vi "函数类型1测试.vi"() -> ()   [LabVIEW 2010]
uses:
  全局量/试验配置信息.vi
panel:
  out "D_IN_1":string[][](table) caption="表格"
  in  "加载文件名称":string
  out "配置文件路径":path
  out "配置文件目录":path
  in  "加载配置文件列表":u16(ring)
  in  "同步_1":i32
  in  "数组_反馈值":dbl[][](array[numeric])
  in  "第几个数据":i32
  in  "第几组数据":i32
  in  "数组_设定值":dbl[][](array[numeric])
  in  "数组_选择":bool[](array[boolean])
  out "light_32":bool
  out "light_31":bool
  out "light_30":bool
  out "light_29":bool
  out "light_28":bool
  out "light_27":bool
  out "light_26":bool
  out "light_25":bool
  out "light_24":bool
  out "light_23":bool
  out "light_22":bool
  out "light_21":bool
  out "light_20":bool
  out "light_19":bool
  out "light_18":bool
  out "light_17":bool
  out "Analog_back":string[][](table) caption="表格"
  in  "A_32":bool
  in  "A_31":bool
  in  "A_30":bool
  in  "A_29":bool
  in  "A_28":bool
  in  "A_27":bool
  in  "A_26":bool
  in  "A_25":bool
  in  "A_24":bool
  in  "A_23":bool
  in  "A_22":bool
  in  "A_21":bool
  in  "A_20":bool
  in  "A_19":bool
  in  "A_18":bool
  in  "A_17":bool
  out "合格？":bool[][](array[boolean])
  out "测试结论":string
  out "light_16":bool
  out "light_15":bool
  out "light_14":bool
  out "light_13":bool
  out "light_12":bool
  out "light_11":bool
  out "light_10":bool
  out "light_9":bool
  out "light_8":bool
  out "light_7":bool
  out "light_6":bool
  out "light_5":bool
  out "light_4":bool
  out "light_3":bool
  out "light_2":bool
  out "light_1":bool
  out "退出？":bool
  in  "btn_反选":bool
  in  "btn_全选":bool
  in  "A_16":bool
  in  "A_15":bool
  in  "A_14":bool
  in  "A_13":bool
  in  "A_12":bool
  in  "A_11":bool
  in  "A_10":bool
  in  "A_9":bool
  in  "A_8":bool
  in  "A_7":bool
  in  "A_6":bool
  in  "A_5":bool
  in  "A_4":bool
  in  "A_3":bool
  in  "A_2":bool
  in  "A_1":bool
  in  "btn_取消":bool
  in  "btn_开始测试":bool
  in  "Analog_IN":string[][](table) caption="表格"
  out "Analog_WC":string[][](table) caption="表格"
  # "模拟量选择及输入值（V）"
  # "模拟量反馈值（V）"
  # "模拟量误差值（%）"
  # "加载配置文件："
  # "测试结论："
  # "从0开始"
  # "从1开始,第0列没有使用"
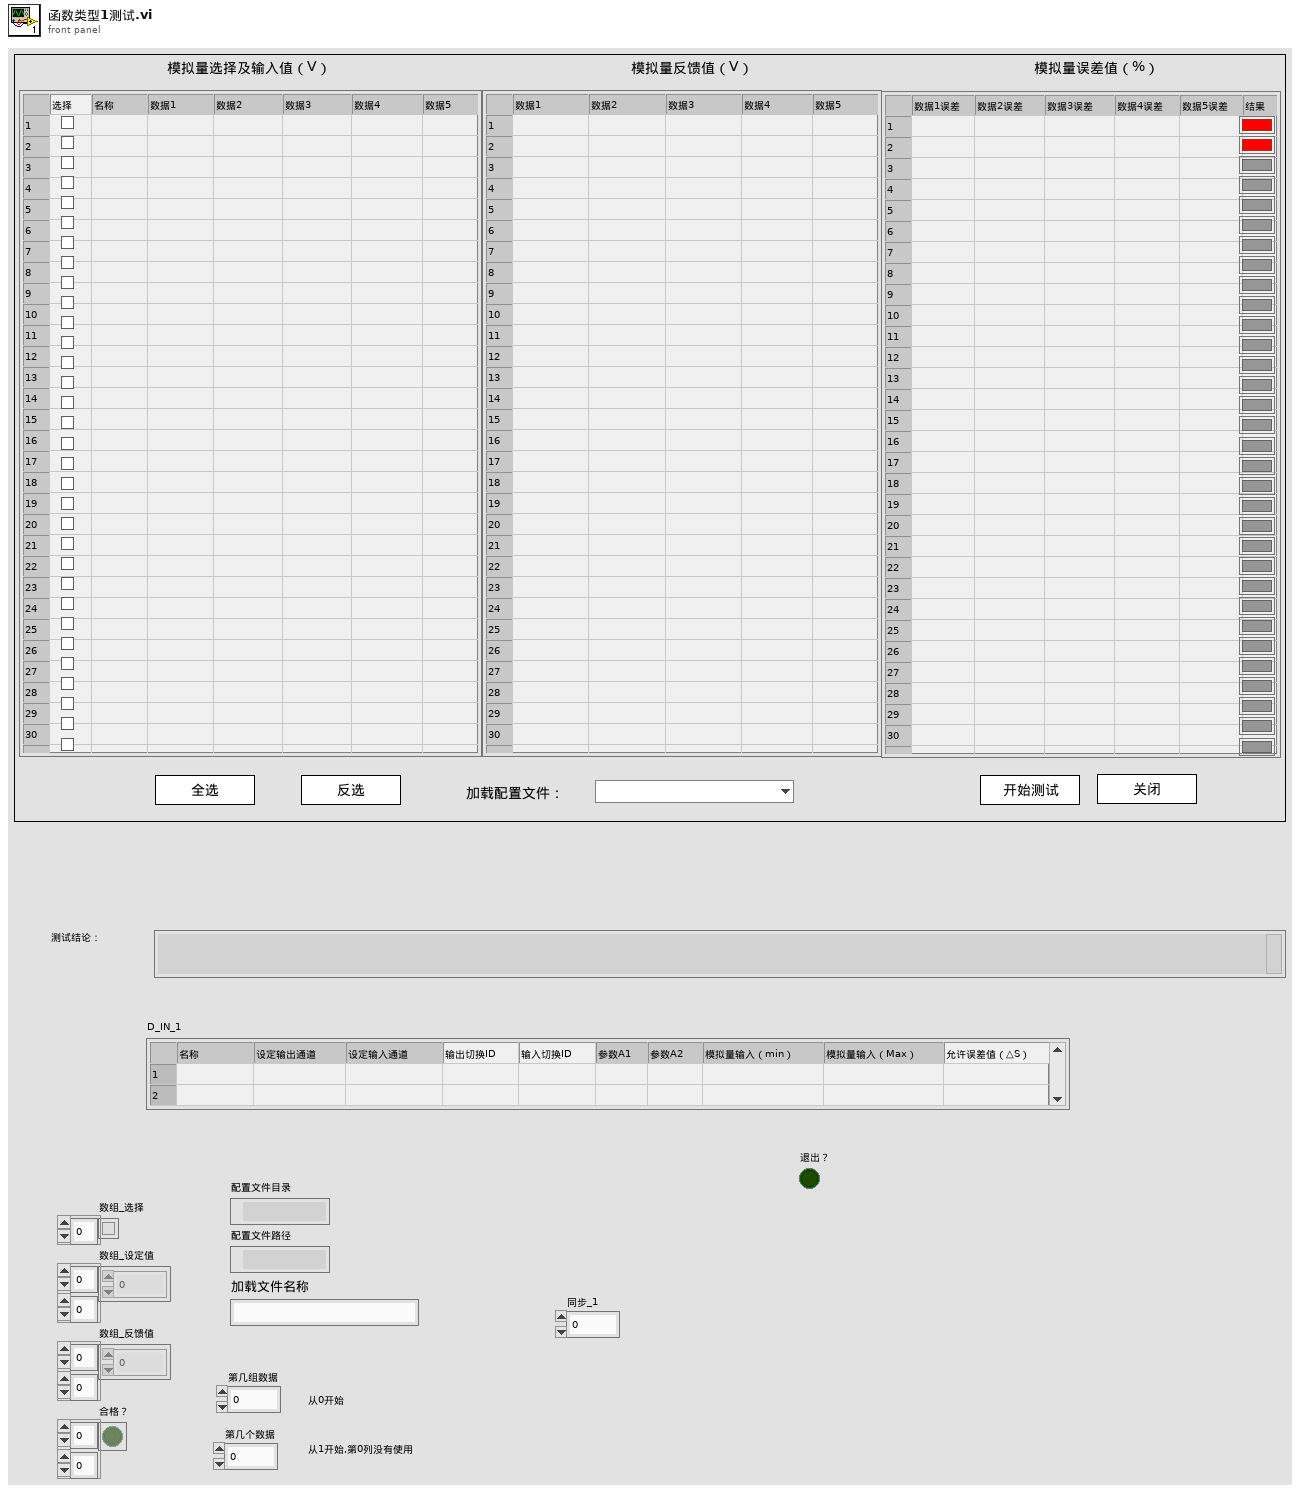
[diagram p1: front panel]
types:
  T1 = enum8{"Enabled", "Disabled", "Disabled and Grayed Out"}
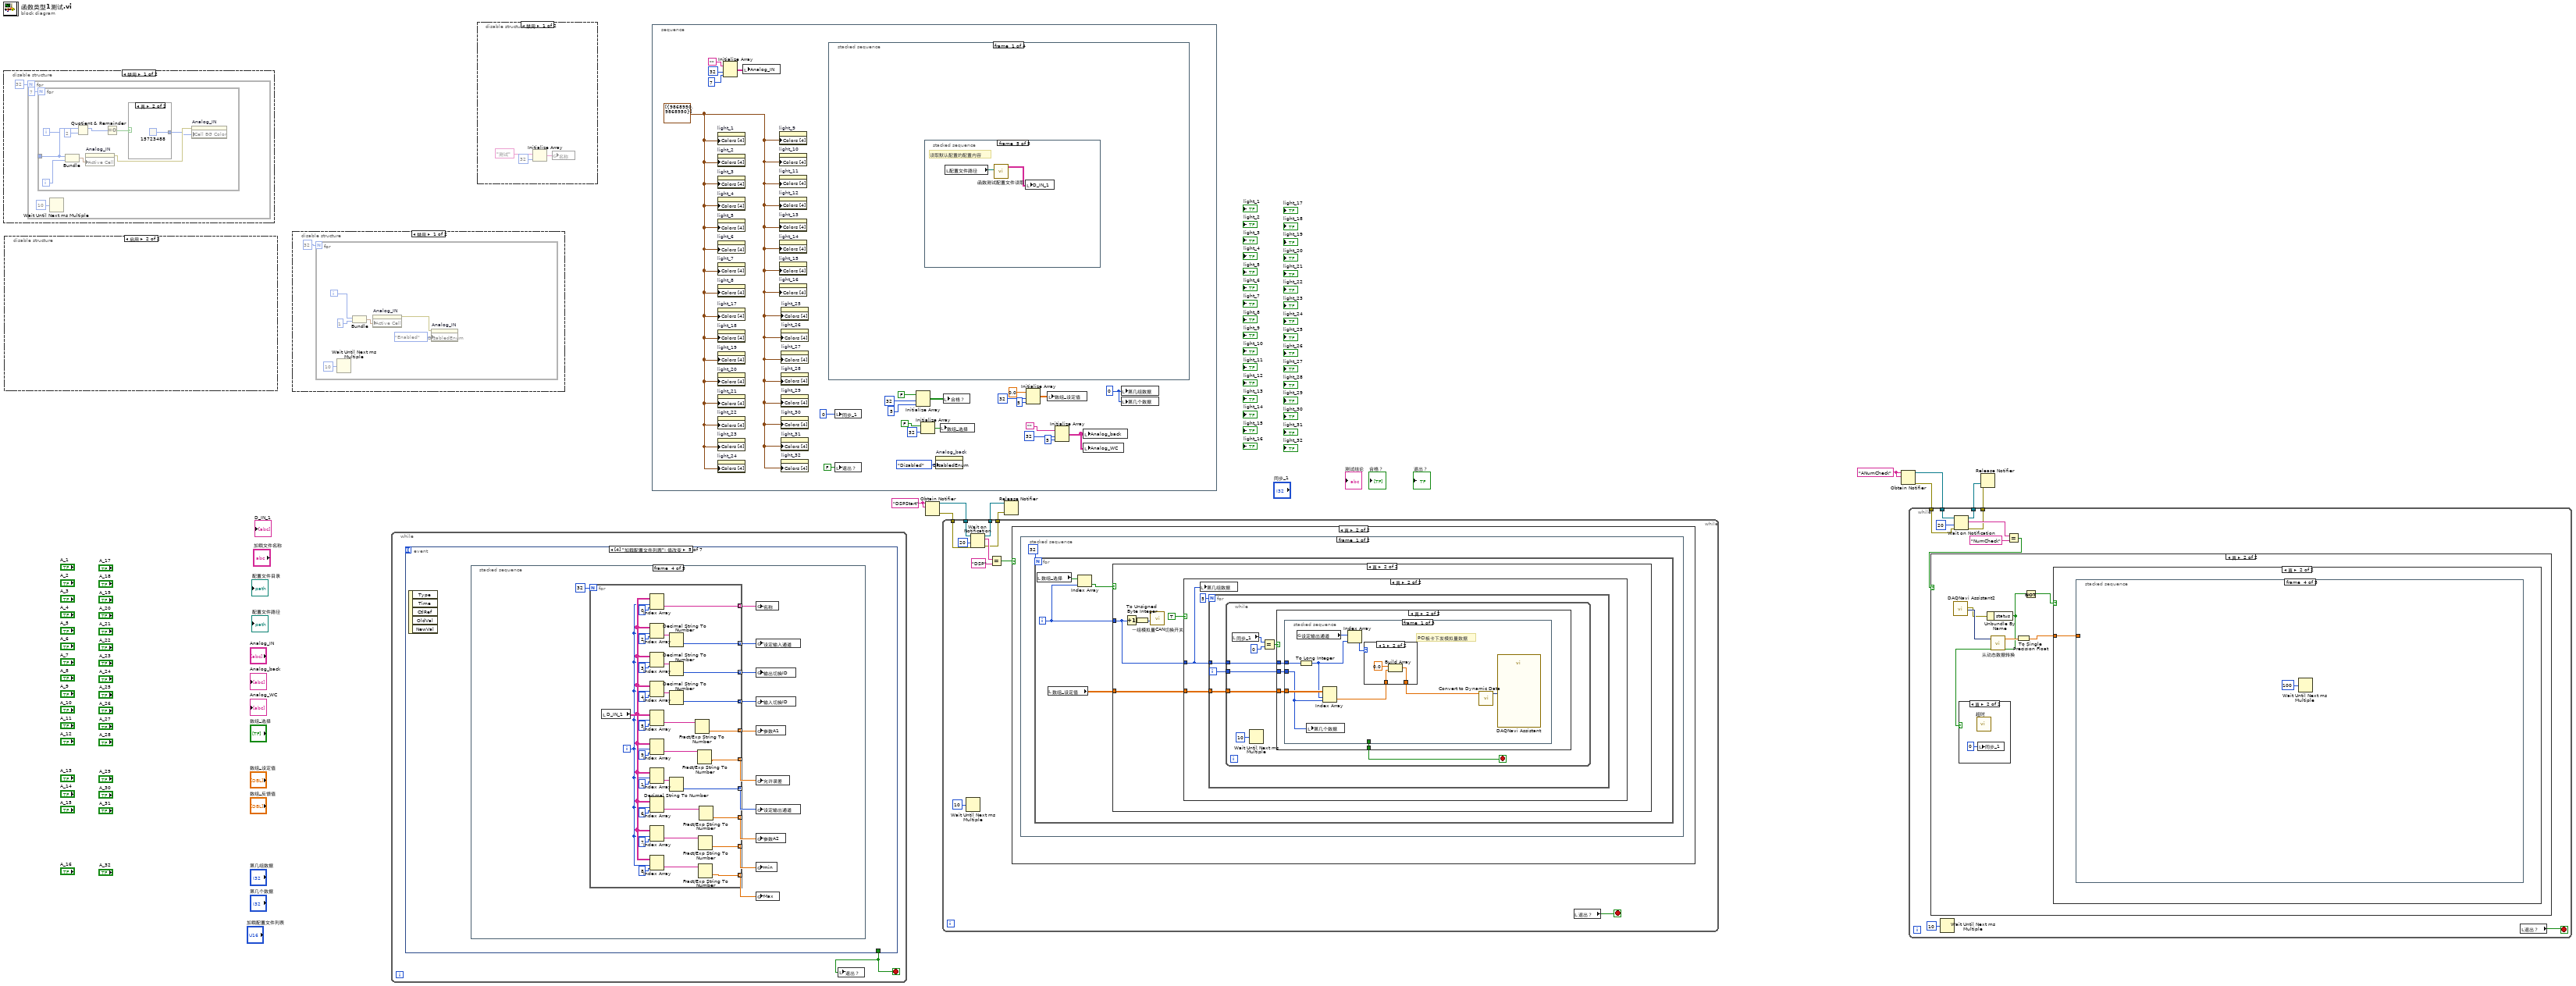
[diagram p0: block diagram]
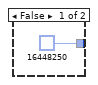
[diagram p3: hidden frame]
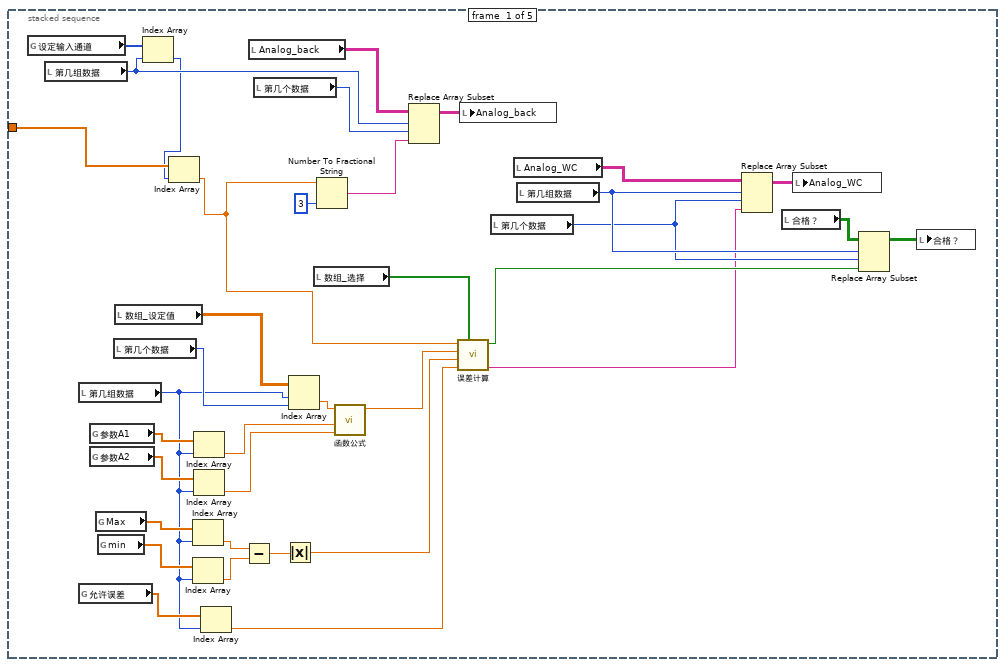
[diagram p8: hidden frame]
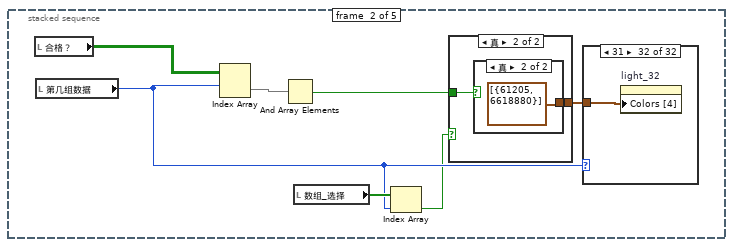
[diagram p9: hidden frame]
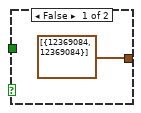
[diagram p10: hidden frame]
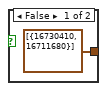
[diagram p11: hidden frame]
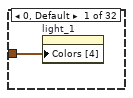
[diagram p12: hidden frame]
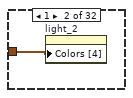
[diagram p13: hidden frame]
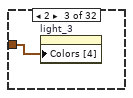
[diagram p14: hidden frame]
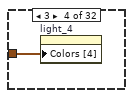
[diagram p15: hidden frame]
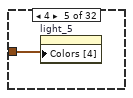
[diagram p16: hidden frame]
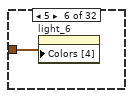
[diagram p17: hidden frame]
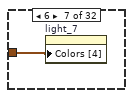
[diagram p18: hidden frame]
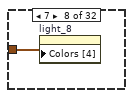
[diagram p19: hidden frame]
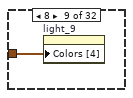
[diagram p20: hidden frame]
diagram:
  w5 = "ANumCheck" ("名称（未命名）")
  w8 = "DSPStart" ("名称（未命名）")
  n1 = disable-structure shown="禁用" {
    frame Disabled {
      n2 = for {
        N: 32 -> [_]
        i -> [w13]
        n3 = for {
          N: 7 -> [_]
          tunnel: w13 -> [w21]
          i -> [w15]
          n4 = Bundle(w21, w15) -> (w18:cluster{i32, i32})  [unwired: 1 in]
          n5 = Quotient & Remainder(x=w21, y=2) -> (x-y*floor(x/y)=w19:i32)  [unwired: 1 out]
          n6 = property on="Analog_IN" class="Tbl (严格)"("Active Cell"=w18) -> (error out=w17:errorcluster)  [unwired: 2 in, 1 out]
          n7 = Equal To 0?(x=w19) -> (x = 0?=w22:bool)
          n8 = case shown="真" w22 {
            tunnel: [u32 16448250 u32 15723488] -> w16
            frame False {
            }
            frame True {
            }
          }
          n9 = property on="Analog_IN" class="Tbl (严格)"(error in=w17, "Cell BG Color"=w16) -> ()  [unwired: 1 in, 2 out]
        }
        n10 = Wait Until Next ms Multiple(millisecond multiple=u32 10 ("毫秒倍数")) -> ()  [unwired: 1 out]
      }
    }
    frame Enabled {
    }
  }
  n11 = disable-structure shown="启用" {
    frame Disabled {
      n12 = for {
        N: 32 -> [_]
        i -> [w26]
        n13 = for {
          N: 7 -> [_]
          tunnel: w26 -> [w29]
          i -> [w30]
          n14 = Bundle(w29, w30) -> (w33:cluster{i32, i32})  [unwired: 1 in]
          n15 = property on="Analog_IN" class="Tbl (严格)"("Active Cell"=w33) -> (error out=w31:errorcluster)  [unwired: 2 in, 1 out]
          n16 = property on="Analog_IN" class="Tbl (严格)"(error in=w31, "Justify"=enum16{"Left", "Center", "Right"}."Left" ("活动单元格:单元格对齐")) -> ()  [unwired: 1 in, 2 out]
        }
        n17 = Wait Until Next ms Multiple(millisecond multiple=u32 10 ("毫秒倍数")) -> ()  [unwired: 1 out]
      }
    }
    frame Enabled {
    }
  }
  n18 = disable-structure shown="禁用" {
    frame Disabled {
      n19 = for {
        N: 32 -> [_]
        i -> [w39]
        n20 = Wait Until Next ms Multiple(millisecond multiple=u32 10 ("毫秒倍数")) -> ()  [unwired: 1 out]
        n21 = Bundle(w39, 1) -> (w38:cluster{i32, i32})  [unwired: 1 in]
        n22 = property on="Analog_IN" class="Tbl (严格)"("Active Cell"=w38) -> (error out=w35:errorcluster)  [unwired: 2 in, 1 out]
        n23 = property on="Analog_IN" class="Tbl (严格)"(error in=w35, "DisabledEnum"=T1."Enabled" ("禁用")) -> ()  [unwired: 1 in, 2 out]
      }
    }
    frame Enabled {
    }
  }
  n24 = while {
    stop <- w41 stop-if-true
    n25 = event shown="[4] \"加载配置文件列表\": 值改变" {
      selector: _ -> [_ _ _ _ _ _ _]
      dyn-events: _ -> [_ _ _ _ _ _ _]
      timeout: _ -> [_ _ _ _ _ _ _]
      tunnel: [_ TRUE TRUE _ _ _ _] -> w41
      event Timeout {
        n26 = event-data() -> ()  [unwired: 1 in, 2 out]
      }
      event Panel Close {
        n27 = event-data() -> ()  [unwired: 1 in, 3 out]
      }
      event "btn_取消": Value Change {
        n28 = event-data() -> ()  [unwired: 1 in, 5 out]
      }
      event "btn_开始测试": Value Change {
        n29 = event-data() -> ()  [unwired: 1 in, 5 out]
        n30 = stacked-sequence {
          frame #0 {
            w49 = 0 ("第几组数据")
            # "测试期间不准退出防止程序卡死"
            n31 = local read "Analog_IN"() -> (w55:string[][])
            n32 = Delete From Array(array=w55, length=1 ("长度"), index (col)=0 ("禁用的索引 (列)")) -> (array with subset deleted=w47:string[][])  [unwired: 1 in, 1 out]
            n33 = Delete From Array(array=w47, length=1 ("长度"), index (col)=0 ("禁用的索引 (列)")) -> (array with subset deleted=w45:string[][])  [unwired: 1 in, 1 out]
            n34 = for {
              N: 32 -> [_]
              tunnel: w45 -> [w58] mode=indexing
              tunnel: [w57] -> w54 mode=indexing
              n35 = for {
                N: 5 -> [_]
                tunnel: w58 -> [w60] mode=indexing
                tunnel: [w59] -> w57 mode=indexing
                n36 = Fract/Exp String To Number(string=w60) -> (number=w59:dbl)  [unwired: 3 in, 1 out]
              }
            }
            n37 = local write "第几组数据"(w49) -> ()
            n38 = local write "第几个数据"(w49) -> ()
            n39 = local write "同步_1"(0 ("同步_2")) -> ()
            n40 = property on="btn_取消" class="Bool"("DisabledEnum"=T1."Disabled and Grayed Out" ("禁用")) -> ()  [unwired: 2 in, 2 out]
            n41 = local write "数组_设定值"(w54) -> ()
          }
          frame #1 {
            n42 = local read "Analog_back"() -> (w63:string[][])
            n43 = local read "Analog_WC"() -> (w62:string[][])
            n44 = for {
              tunnel: w62 -> [w99] mode=indexing
              i -> [w98]
              n45 = for {
                tunnel: w99 -> [_] mode=indexing
                tunnel: w98 -> [w103]
                i -> [w102]
                n46 = local read "Analog_WC"() -> (w104:string[][])
                n47 = Replace Array Subset(array=w104, new element="", index (row)=w103, index (col)=w102) -> (w100:string[][])
                n48 = local write "Analog_WC"(w100) -> ()
              }
            }
            n49 = for {
              tunnel: w63 -> [w106] mode=indexing
              i -> [w105]
              n50 = for {
                tunnel: w106 -> [_] mode=indexing
                tunnel: w105 -> [w110]
                i -> [w109]
                n51 = local read "Analog_back"() -> (w111:string[][])
                n52 = Replace Array Subset(array=w111, new element="", index (row)=w110, index (col)=w109) -> (w107:string[][])
                n53 = local write "Analog_back"(w107) -> ()
              }
            }
            n54 = for {
              N: 32 -> [_]
              i -> [w65]
              n55 = case shown="31" w65 {
                tunnel: cluster{u32, u32}[] [{9868950, 9868950}] -> [w66 w67 w68 w69 w70 w71 w72 w73 w74 w75 w76 w77 w78 w79 w80 w81 w82 w83 w84 w85 w86 w87 w88 w89 w90 w91 w92 w93 w94 w95 w96 w97]
                frame 0, Default {
                  n56 = property on="light_1" class="Bool (严格)"("Colors [4]"=w66) -> ()  [unwired: 2 in, 2 out]
                }
                frame 1 {
                  n57 = property on="light_2" class="Bool (严格)"("Colors [4]"=w67) -> ()  [unwired: 2 in, 2 out]
                }
                frame 2 {
                  n58 = property on="light_3" class="Bool (严格)"("Colors [4]"=w68) -> ()  [unwired: 2 in, 2 out]
                }
                frame 3 {
                  n59 = property on="light_4" class="Bool (严格)"("Colors [4]"=w69) -> ()  [unwired: 2 in, 2 out]
                }
                frame 4 {
                  n60 = property on="light_5" class="Bool (严格)"("Colors [4]"=w70) -> ()  [unwired: 2 in, 2 out]
                }
                frame 5 {
                  n61 = property on="light_6" class="Bool (严格)"("Colors [4]"=w71) -> ()  [unwired: 2 in, 2 out]
                }
                frame 6 {
                  n62 = property on="light_7" class="Bool (严格)"("Colors [4]"=w72) -> ()  [unwired: 2 in, 2 out]
                }
                frame 7 {
                  n63 = property on="light_8" class="Bool (严格)"("Colors [4]"=w73) -> ()  [unwired: 2 in, 2 out]
                }
                frame 8 {
                  n64 = property on="light_9" class="Bool (严格)"("Colors [4]"=w74) -> ()  [unwired: 2 in, 2 out]
                }
                frame 9 {
                  n65 = property on="light_10" class="Bool (严格)"("Colors [4]"=w75) -> ()  [unwired: 2 in, 2 out]
                }
                frame 10 {
                  n66 = property on="light_11" class="Bool (严格)"("Colors [4]"=w76) -> ()  [unwired: 2 in, 2 out]
                }
                frame 11 {
                  n67 = property on="light_12" class="Bool (严格)"("Colors [4]"=w77) -> ()  [unwired: 2 in, 2 out]
                }
                frame 12 {
                  n68 = property on="light_13" class="Bool (严格)"("Colors [4]"=w78) -> ()  [unwired: 2 in, 2 out]
                }
                frame 13 {
                  n69 = property on="light_14" class="Bool (严格)"("Colors [4]"=w79) -> ()  [unwired: 2 in, 2 out]
                }
                frame 14 {
                  n70 = property on="light_15" class="Bool (严格)"("Colors [4]"=w80) -> ()  [unwired: 2 in, 2 out]
                }
                frame 15 {
                  n71 = property on="light_16" class="Bool (严格)"("Colors [4]"=w81) -> ()  [unwired: 2 in, 2 out]
                }
                frame 16 {
                  n72 = property on="light_17" class="Bool (严格)"("Colors [4]"=w82) -> ()  [unwired: 2 in, 2 out]
                }
                frame 17 {
                  n73 = property on="light_18" class="Bool (严格)"("Colors [4]"=w83) -> ()  [unwired: 2 in, 2 out]
                }
                frame 18 {
                  n74 = property on="light_19" class="Bool (严格)"("Colors [4]"=w84) -> ()  [unwired: 2 in, 2 out]
                }
                frame 19 {
                  n75 = property on="light_20" class="Bool (严格)"("Colors [4]"=w85) -> ()  [unwired: 2 in, 2 out]
                }
                frame 20 {
                  n76 = property on="light_21" class="Bool (严格)"("Colors [4]"=w86) -> ()  [unwired: 2 in, 2 out]
                }
                frame 21 {
                  n77 = property on="light_22" class="Bool (严格)"("Colors [4]"=w87) -> ()  [unwired: 2 in, 2 out]
                }
                frame 22 {
                  n78 = property on="light_23" class="Bool (严格)"("Colors [4]"=w88) -> ()  [unwired: 2 in, 2 out]
                }
                frame 23 {
                  n79 = property on="light_24" class="Bool (严格)"("Colors [4]"=w89) -> ()  [unwired: 2 in, 2 out]
                }
                frame 24 {
                  n80 = property on="light_25" class="Bool (严格)"("Colors [4]"=w90) -> ()  [unwired: 2 in, 2 out]
                }
                frame 25 {
                  n81 = property on="light_26" class="Bool (严格)"("Colors [4]"=w91) -> ()  [unwired: 2 in, 2 out]
                }
                frame 26 {
                  n82 = property on="light_27" class="Bool (严格)"("Colors [4]"=w92) -> ()  [unwired: 2 in, 2 out]
                }
                frame 27 {
                  n83 = property on="light_28" class="Bool (严格)"("Colors [4]"=w93) -> ()  [unwired: 2 in, 2 out]
                }
                frame 28 {
                  n84 = property on="light_29" class="Bool (严格)"("Colors [4]"=w94) -> ()  [unwired: 2 in, 2 out]
                }
                frame 29 {
                  n85 = property on="light_30" class="Bool (严格)"("Colors [4]"=w95) -> ()  [unwired: 2 in, 2 out]
                }
                frame 30 {
                  n86 = property on="light_31" class="Bool (严格)"("Colors [4]"=w96) -> ()  [unwired: 2 in, 2 out]
                }
                frame 31 {
                  n87 = property on="light_32" class="Bool (严格)"("Colors [4]"=w97) -> ()  [unwired: 2 in, 2 out]
                }
              }
            }
          }
          frame #2 {
            n88 = for {
              N: 32 -> [_]
              i -> [w114]
              n89 = disable-structure shown="禁用" {
                frame Disabled {
                  n90 = Wait Until Next ms Multiple(millisecond multiple=u32 10 ("毫秒倍数")) -> ()  [unwired: 1 out]
                }
                frame Enabled {
                }
              }
              n91 = for {
                N: 6 -> [_]
                tunnel: w114 -> [w122]
                i -> [w119]
                n92 = Quotient & Remainder(x=w122, y=2) -> (x-y*floor(x/y)=w120:i32)  [unwired: 1 out]
                n93 = Equal To 0?(x=w120) -> (x = 0?=w123:bool)
                n94 = case shown="假" w123 {
                  tunnel: [u32 16448250 u32 15723488] -> w116
                  frame False {
                  }
                  frame True {
                  }
                }
                n95 = Bundle(w122, w119) -> (w118:cluster{i32, i32})  [unwired: 1 in]
                n96 = property on="Analog_WC" class="Tbl (严格)"("Active Cell"=w118) -> (error out=w117:errorcluster)  [unwired: 2 in, 1 out]
                n97 = property on="Analog_WC" class="Tbl (严格)"(error in=w117, "Cell BG Color"=w116) -> ()  [unwired: 1 in, 2 out]
              }
            }
          }
          frame #3 {
            n98 = local read "A_10"() -> (w154:bool)
            n99 = local read "A_11"() -> (w153:bool)
            n100 = local read "A_12"() -> (w152:bool)
            n101 = local read "A_13"() -> (w151:bool)
            n102 = local read "A_14"() -> (w150:bool)
            n103 = local read "A_15"() -> (w149:bool)
            n104 = local read "A_16"() -> (w148:bool)
            n105 = local read "A_17"() -> (w147:bool)
            n106 = local read "A_18"() -> (w146:bool)
            n107 = local read "A_19"() -> (w145:bool)
            n108 = local read "A_20"() -> (w144:bool)
            n109 = local read "A_21"() -> (w143:bool)
            n110 = local read "A_22"() -> (w142:bool)
            n111 = local read "A_23"() -> (w141:bool)
            n112 = local read "A_24"() -> (w140:bool)
            n113 = local read "A_25"() -> (w139:bool)
            n114 = local read "A_26"() -> (w138:bool)
            n115 = local read "A_27"() -> (w137:bool)
            n116 = local read "A_28"() -> (w136:bool)
            n117 = local read "A_29"() -> (w135:bool)
            n118 = local read "A_30"() -> (w134:bool)
            n119 = local read "A_31"() -> (w133:bool)
            n120 = local read "A_32"() -> (w132:bool)
            n121 = local read "A_1"() -> (w163:bool)
            n122 = local read "A_2"() -> (w162:bool)
            n123 = local read "A_3"() -> (w161:bool)
            n124 = local read "A_4"() -> (w160:bool)
            n125 = local read "A_5"() -> (w159:bool)
            n126 = local read "A_6"() -> (w158:bool)
            n127 = local read "A_7"() -> (w157:bool)
            n128 = local read "A_8"() -> (w156:bool)
            n129 = local read "A_9"() -> (w155:bool)
            n130 = Build Array(w163, w162, w161, w160, w159, w158, w157, w156, w155, w154, w153, w152, w151, w150, w149, w148, w147, w146, w145, w144, w143, w142, w141, w140, w139, w138, w137, w136, w135, w134, w133, w132) -> (w126:bool[])
            n131 = Or Array Elements(Boolean array=w126) -> (logical OR=w131:bool)
            n132 = case shown="真" w131 {
              frame False {
                n133 = call "显示对话框信息"() -> ()  [unwired: 10 in, 2 out]
              }
              frame True {
                w166 = "DSPStart" ("名称（未命名）")
                n134 = Obtain Notifier(name (unnamed)=w166, notification data type=w166) -> (notifier out=w165:refnum<notifier>)  [unwired: 2 in, 2 out]
                n135 = Send Notification(notification="DSP" ("通知"), notifier=w165) -> ()  [unwired: 1 in, 2 out]
              }
            }
            n136 = local write "数组_选择"(w126) -> ()
            n137 = Initialize Array(FALSE, 32 ("维数大小"), 5 ("维数大小")) -> (w127:bool[][])
            n138 = local write "合格？"(w127) -> ()
          }
        }
      }
      event "加载配置文件列表": Value Change {
        n139 = event-data() -> ()  [unwired: 1 in, 5 out]
        n140 = stacked-sequence {
          frame #0 {
            n141 = property on="加载配置文件列表" class="Ring (严格)"() -> ("RingText.Text"=w167:string)  [unwired: 2 in, 2 out]
            n142 = local write "加载文件名称"(w167) -> ()
          }
          frame #1 {
            n143 = local read "配置文件目录"() -> (w170:path)
            n144 = property on="加载文件名称" class="Str"() -> ("Text.Text"=w168:string)  [unwired: 2 in, 2 out]
            n145 = Build Path(base path=w170, name or relative path=w168) -> (appended path=w169:path)
            n146 = local write "配置文件路径"(w169) -> ()
          }
          frame #2 {
            n147 = local read "配置文件路径"() -> (w172:path)
            n148 = call "函数测试配置文件读取.vi"("配置文件路径"=w172) -> ("D_IN_1"=w171:string[][])  [unwired: 6 in, 3 out]
            n149 = local write "D_IN_1"(w171) -> ()
          }
          frame #3 {
            n150 = for {
              N: 32 ("维数大小") -> [_]
              tunnel: [w213] -> w178 mode=indexing
              tunnel: [w188] -> w177 mode=indexing
              tunnel: [w208] -> w176 mode=indexing
              tunnel: [w205] -> w175 mode=indexing
              tunnel: [w202] -> w180 mode=indexing
              tunnel: [w199] -> w181 mode=indexing
              tunnel: [w186] -> w182 mode=indexing
              tunnel: [w190] -> w174 mode=indexing
              tunnel: [w184] -> w183 mode=indexing
              tunnel: [w192] -> w173 mode=indexing
              i -> [w194]
              n151 = local read "D_IN_1"() -> (w195:string[][])
              n152 = Index Array(array=w195, index (row)=w194, index (col)=0 ("禁用的索引 (列)")) -> (element=w213:string)
              n153 = Index Array(array=w195, index (row)=w194, index (col)=2 ("禁用的索引 (列)")) -> (element=w207:string)
              n154 = Index Array(array=w195, index (row)=w194, index (col)=3 ("禁用的索引 (列)")) -> (element=w203:string)
              n155 = Index Array(array=w195, index (row)=w194, index (col)=4 ("禁用的索引 (列)")) -> (element=w201:string)
              n156 = Index Array(array=w195, index (row)=w194, index (col)=5 ("禁用的索引 (列)")) -> (element=w187:string)
              n157 = Index Array(array=w195, index (row)=w194, index (col)=9 ("禁用的索引 (列)")) -> (element=w185:string)
              n158 = Index Array(array=w195, index (row)=w194, index (col)=1 ("禁用的索引 (列)")) -> (element=w210:string)
              n159 = Index Array(array=w195, index (row)=w194, index (col)=6 ("禁用的索引 (列)")) -> (element=w191:string)
              n160 = Index Array(array=w195, index (row)=w194, index (col)=7 ("禁用的索引 (列)")) -> (element=w193:string)
              n161 = Index Array(array=w195, index (row)=w194, index (col)=8 ("禁用的索引 (列)")) -> (element=w189:string)
              n162 = Decimal String To Number(string=w207) -> (number=w205:i32)  [unwired: 2 in, 1 out]
              n163 = Decimal String To Number(string=w203) -> (number=w202:i32)  [unwired: 2 in, 1 out]
              n164 = Decimal String To Number(string=w201) -> (number=w199:i32)  [unwired: 2 in, 1 out]
              n165 = Decimal String To Number(string=w210) -> (number=w208:i32)  [unwired: 2 in, 1 out]
              n166 = Fract/Exp String To Number(string=w187) -> (number=w186:dbl)  [unwired: 3 in, 1 out]
              n167 = Fract/Exp String To Number(string=w185) -> (number=w184:dbl)  [unwired: 3 in, 1 out]
              n168 = Fract/Exp String To Number(string=w193) -> (number=w192:dbl)  [unwired: 3 in, 1 out]
              n169 = Fract/Exp String To Number(string=w189) -> (number=w188:dbl)  [unwired: 3 in, 1 out]
              n170 = Fract/Exp String To Number(string=w191) -> (number=w190:dbl)  [unwired: 3 in, 1 out]
            }
            n171 = global write "试验配置信息.vi" "名称"(w178) -> ()
            n172 = global write "试验配置信息.vi" "设定输入通道"(w175) -> ()
            n173 = global write "试验配置信息.vi" "输出切换ID"(w180) -> ()
            n174 = global write "试验配置信息.vi" "输入切换ID"(w181) -> ()
            n175 = global write "试验配置信息.vi" "参数A1"(w182) -> ()
            n176 = global write "试验配置信息.vi" "允许误差"(w183) -> ()
            n177 = global write "试验配置信息.vi" "设定输出通道"(w176) -> ()
            n178 = global write "试验配置信息.vi" "参数A2"(w174) -> ()
            n179 = global write "试验配置信息.vi" "min"(w173) -> ()
            n180 = global write "试验配置信息.vi" "Max"(w177) -> ()
          }
          frame #4 {
            n181 = for {
              N: 32 -> [_]
              i -> [w218]
              w222 = 5 ("num")
              n182 = global read "试验配置信息.vi" "名称"() -> (w221:string[])
              n183 = global read "试验配置信息.vi" "Max"() -> (w225:dbl[])
              n184 = global read "试验配置信息.vi" "min"() -> (w226:dbl[])
              n185 = Index Array(array=w226, index=w218) -> (element=w224:dbl)
              n186 = Index Array(array=w225, index=w218) -> (element=w223:dbl)
              n187 = for {
                N: w222 -> [_]
                tunnel: w218 -> [w237]
                tunnel: w224 -> [w234]
                tunnel: w223 -> [w233]
                tunnel: w222 -> [w232]
                i -> [w230]
                n188 = call "等分取数据.vi"("Max"=w233, "MIN"=w234, "num"=w232) -> ("数据点"=w231:dbl[])  [unwired: 5 in]
                n189 = Add(x=2, y=w230) -> (x+y=w235:i32)
                n190 = local read "Analog_IN"() -> (w239:string[][])
                n191 = Index Array(array=w231, index=w230) -> (element=w228:dbl)
                n192 = Number To Fractional String(number=w228, precision (6)=i16 3 ("精度(6)")) -> (F-format string=w227:string)  [unwired: 2 in]
                n193 = Replace Array Subset(array=w239, new element=w227, index (row)=w237, index (col)=w235) -> (w238:string[][])
                n194 = local write "Analog_IN"(w238) -> ()
              }
              n195 = Index Array(array=w221, index=w218) -> (element=w216:string)
              n196 = local read "Analog_IN"() -> (w219:string[][])
              n197 = Replace Array Subset(array=w219, new element=w216, index (row)=w218, index (col)=1) -> (w220:string[][])
              n198 = local write "Analog_IN"(w220) -> ()
            }
          }
        }
      }
      event "btn_全选": Value Change {
        w240 = TRUE ("单选_AD_1")
        n199 = event-data() -> ()  [unwired: 1 in, 5 out]
        n200 = local write "A_1"(w240) -> ()
        n201 = local write "A_2"(w240) -> ()
        n202 = local write "A_3"(w240) -> ()
        n203 = local write "A_4"(w240) -> ()
        n204 = local write "A_5"(w240) -> ()
        n205 = local write "A_6"(w240) -> ()
        n206 = local write "A_7"(w240) -> ()
        n207 = local write "A_8"(w240) -> ()
        n208 = local write "A_9"(w240) -> ()
        n209 = local write "A_10"(w240) -> ()
        n210 = local write "A_11"(w240) -> ()
        n211 = local write "A_12"(w240) -> ()
        n212 = local write "A_13"(w240) -> ()
        n213 = local write "A_14"(w240) -> ()
        n214 = local write "A_15"(w240) -> ()
        n215 = local write "A_16"(w240) -> ()
        n216 = local write "A_17"(w240) -> ()
        n217 = local write "A_18"(w240) -> ()
        n218 = local write "A_19"(w240) -> ()
        n219 = local write "A_20"(w240) -> ()
        n220 = local write "A_21"(w240) -> ()
        n221 = local write "A_22"(w240) -> ()
        n222 = local write "A_23"(w240) -> ()
        n223 = local write "A_24"(w240) -> ()
        n224 = local write "A_25"(w240) -> ()
        n225 = local write "A_26"(w240) -> ()
        n226 = local write "A_27"(w240) -> ()
        n227 = local write "A_28"(w240) -> ()
        n228 = local write "A_29"(w240) -> ()
        n229 = local write "A_30"(w240) -> ()
        n230 = local write "A_31"(w240) -> ()
        n231 = local write "A_32"(w240) -> ()
      }
      event "btn_反选": Value Change {
        n232 = event-data() -> ()  [unwired: 1 in, 5 out]
        n233 = local read "A_17"() -> (w272:bool)
        n234 = local read "A_18"() -> (w270:bool)
        n235 = local read "A_19"() -> (w268:bool)
        n236 = local read "A_20"() -> (w266:bool)
        n237 = local read "A_21"() -> (w264:bool)
        n238 = local read "A_22"() -> (w262:bool)
        n239 = local read "A_23"() -> (w260:bool)
        n240 = local read "A_24"() -> (w258:bool)
        n241 = local read "A_25"() -> (w256:bool)
        n242 = local read "A_26"() -> (w254:bool)
        n243 = local read "A_27"() -> (w252:bool)
        n244 = local read "A_28"() -> (w250:bool)
        n245 = local read "A_29"() -> (w248:bool)
        n246 = local read "A_30"() -> (w246:bool)
        n247 = local read "A_31"() -> (w244:bool)
        n248 = local read "A_32"() -> (w242:bool)
        n249 = local read "A_1"() -> (w304:bool)
        n250 = local read "A_2"() -> (w302:bool)
        n251 = local read "A_3"() -> (w301:bool)
        n252 = local read "A_4"() -> (w300:bool)
        n253 = local read "A_5"() -> (w299:bool)
        n254 = local read "A_6"() -> (w298:bool)
        n255 = local read "A_7"() -> (w297:bool)
        n256 = local read "A_8"() -> (w296:bool)
        n257 = local read "A_9"() -> (w295:bool)
        n258 = local read "A_10"() -> (w294:bool)
        n259 = local read "A_11"() -> (w293:bool)
        n260 = local read "A_12"() -> (w292:bool)
        n261 = local read "A_13"() -> (w291:bool)
        n262 = local read "A_14"() -> (w290:bool)
        n263 = local read "A_15"() -> (w289:bool)
        n264 = local read "A_16"() -> (w288:bool)
        n265 = Not(x=w304) -> (.not. x?=w303:bool)
        n266 = Not(x=w302) -> (.not. x?=w273:bool)
        n267 = Not(x=w301) -> (.not. x?=w274:bool)
        n268 = Not(x=w300) -> (.not. x?=w275:bool)
        n269 = Not(x=w299) -> (.not. x?=w276:bool)
        n270 = Not(x=w298) -> (.not. x?=w277:bool)
        n271 = Not(x=w297) -> (.not. x?=w278:bool)
        n272 = Not(x=w296) -> (.not. x?=w279:bool)
        n273 = Not(x=w295) -> (.not. x?=w280:bool)
        n274 = Not(x=w294) -> (.not. x?=w281:bool)
        n275 = Not(x=w293) -> (.not. x?=w282:bool)
        n276 = Not(x=w292) -> (.not. x?=w283:bool)
        n277 = Not(x=w291) -> (.not. x?=w284:bool)
        n278 = Not(x=w290) -> (.not. x?=w285:bool)
        n279 = Not(x=w289) -> (.not. x?=w286:bool)
        n280 = Not(x=w288) -> (.not. x?=w287:bool)
        n281 = Not(x=w272) -> (.not. x?=w271:bool)
        n282 = Not(x=w270) -> (.not. x?=w269:bool)
        n283 = Not(x=w268) -> (.not. x?=w267:bool)
        n284 = Not(x=w266) -> (.not. x?=w265:bool)
        n285 = Not(x=w264) -> (.not. x?=w263:bool)
        n286 = Not(x=w262) -> (.not. x?=w261:bool)
        n287 = Not(x=w260) -> (.not. x?=w259:bool)
        n288 = Not(x=w258) -> (.not. x?=w257:bool)
        n289 = Not(x=w256) -> (.not. x?=w255:bool)
        n290 = Not(x=w254) -> (.not. x?=w253:bool)
        n291 = Not(x=w252) -> (.not. x?=w251:bool)
        n292 = Not(x=w250) -> (.not. x?=w249:bool)
        n293 = Not(x=w248) -> (.not. x?=w247:bool)
        n294 = Not(x=w246) -> (.not. x?=w245:bool)
        n295 = Not(x=w244) -> (.not. x?=w243:bool)
        n296 = Not(x=w242) -> (.not. x?=w241:bool)
        n297 = local write "A_1"(w303) -> ()
        n298 = local write "A_2"(w273) -> ()
        n299 = local write "A_3"(w274) -> ()
        n300 = local write "A_4"(w275) -> ()
        n301 = local write "A_5"(w276) -> ()
        n302 = local write "A_6"(w277) -> ()
        n303 = local write "A_7"(w278) -> ()
        n304 = local write "A_8"(w279) -> ()
        n305 = local write "A_9"(w280) -> ()
        n306 = local write "A_10"(w281) -> ()
        n307 = local write "A_11"(w282) -> ()
        n308 = local write "A_12"(w283) -> ()
        n309 = local write "A_13"(w284) -> ()
        n310 = local write "A_14"(w285) -> ()
        n311 = local write "A_15"(w286) -> ()
        n312 = local write "A_16"(w287) -> ()
        n313 = local write "A_17"(w271) -> ()
        n314 = local write "A_18"(w269) -> ()
        n315 = local write "A_19"(w267) -> ()
        n316 = local write "A_20"(w265) -> ()
        n317 = local write "A_21"(w263) -> ()
        n318 = local write "A_22"(w261) -> ()
        n319 = local write "A_23"(w259) -> ()
        n320 = local write "A_24"(w257) -> ()
        n321 = local write "A_25"(w255) -> ()
        n322 = local write "A_26"(w253) -> ()
        n323 = local write "A_27"(w251) -> ()
        n324 = local write "A_28"(w249) -> ()
        n325 = local write "A_29"(w247) -> ()
        n326 = local write "A_30"(w245) -> ()
        n327 = local write "A_31"(w243) -> ()
        n328 = local write "A_32"(w241) -> ()
      }
    }
    n329 = local write "退出？"(w41) -> ()
  }
  n330 = disable-structure shown="禁用" {
    frame Disabled {
      n331 = Initialize Array("测试", 32 ("维数大小")) -> (w306:string[])
      n332 = global write "试验配置信息.vi" "名称"(w306) -> ()
    }
    frame Enabled {
    }
  }
  n333 = stacked-sequence {
    frame #0 {
      w312 = 0 ("第几组数据")
      w327 = cluster{u32, u32}[] [{9868950, 9868950}]
      n334 = property on="light_1" class="Bool (严格)"("Colors [4]"=w327) -> ()  [unwired: 2 in, 2 out]
      n335 = property on="light_2" class="Bool (严格)"("Colors [4]"=w327) -> ()  [unwired: 2 in, 2 out]
      n336 = property on="light_3" class="Bool (严格)"("Colors [4]"=w327) -> ()  [unwired: 2 in, 2 out]
      n337 = property on="light_4" class="Bool (严格)"("Colors [4]"=w327) -> ()  [unwired: 2 in, 2 out]
      n338 = property on="light_5" class="Bool (严格)"("Colors [4]"=w327) -> ()  [unwired: 2 in, 2 out]
      n339 = property on="light_6" class="Bool (严格)"("Colors [4]"=w327) -> ()  [unwired: 2 in, 2 out]
      n340 = property on="light_7" class="Bool (严格)"("Colors [4]"=w327) -> ()  [unwired: 2 in, 2 out]
      n341 = property on="light_8" class="Bool (严格)"("Colors [4]"=w327) -> ()  [unwired: 2 in, 2 out]
      n342 = property on="light_17" class="Bool (严格)"("Colors [4]"=w327) -> ()  [unwired: 2 in, 2 out]
      n343 = property on="light_18" class="Bool (严格)"("Colors [4]"=w327) -> ()  [unwired: 2 in, 2 out]
      n344 = property on="light_19" class="Bool (严格)"("Colors [4]"=w327) -> ()  [unwired: 2 in, 2 out]
      n345 = property on="light_20" class="Bool (严格)"("Colors [4]"=w327) -> ()  [unwired: 2 in, 2 out]
      n346 = property on="light_21" class="Bool (严格)"("Colors [4]"=w327) -> ()  [unwired: 2 in, 2 out]
      n347 = property on="light_22" class="Bool (严格)"("Colors [4]"=w327) -> ()  [unwired: 2 in, 2 out]
      n348 = property on="light_23" class="Bool (严格)"("Colors [4]"=w327) -> ()  [unwired: 2 in, 2 out]
      n349 = property on="light_24" class="Bool (严格)"("Colors [4]"=w327) -> ()  [unwired: 2 in, 2 out]
      n350 = Initialize Array("", 32 ("维数大小"), 7 ("维数大小")) -> (w311:string[][])
      n351 = local write "Analog_IN"(w311) -> ()
      n352 = property on="light_9" class="Bool (严格)"("Colors [4]"=w327) -> ()  [unwired: 2 in, 2 out]
      n353 = property on="light_10" class="Bool (严格)"("Colors [4]"=w327) -> ()  [unwired: 2 in, 2 out]
      n354 = property on="light_11" class="Bool (严格)"("Colors [4]"=w327) -> ()  [unwired: 2 in, 2 out]
      n355 = property on="light_12" class="Bool (严格)"("Colors [4]"=w327) -> ()  [unwired: 2 in, 2 out]
      n356 = property on="light_13" class="Bool (严格)"("Colors [4]"=w327) -> ()  [unwired: 2 in, 2 out]
      n357 = property on="light_14" class="Bool (严格)"("Colors [4]"=w327) -> ()  [unwired: 2 in, 2 out]
      n358 = property on="light_15" class="Bool (严格)"("Colors [4]"=w327) -> ()  [unwired: 2 in, 2 out]
      n359 = property on="light_16" class="Bool (严格)"("Colors [4]"=w327) -> ()  [unwired: 2 in, 2 out]
      n360 = property on="light_25" class="Bool (严格)"("Colors [4]"=w327) -> ()  [unwired: 2 in, 2 out]
      n361 = property on="light_26" class="Bool (严格)"("Colors [4]"=w327) -> ()  [unwired: 2 in, 2 out]
      n362 = property on="light_27" class="Bool (严格)"("Colors [4]"=w327) -> ()  [unwired: 2 in, 2 out]
      n363 = property on="light_28" class="Bool (严格)"("Colors [4]"=w327) -> ()  [unwired: 2 in, 2 out]
      n364 = property on="light_29" class="Bool (严格)"("Colors [4]"=w327) -> ()  [unwired: 2 in, 2 out]
      n365 = property on="light_30" class="Bool (严格)"("Colors [4]"=w327) -> ()  [unwired: 2 in, 2 out]
      n366 = property on="light_31" class="Bool (严格)"("Colors [4]"=w327) -> ()  [unwired: 2 in, 2 out]
      n367 = property on="light_32" class="Bool (严格)"("Colors [4]"=w327) -> ()  [unwired: 2 in, 2 out]
      n368 = stacked-sequence {
        frame #0 {
          n369 = stacked-sequence {
            frame #0 {
              # "初始化配置文件路径"
              n370 = VI Library "VI库"() -> (path=w337:path)
              n371 = Strip Path(path=w337) -> (stripped path=w336:path)  [unwired: 1 out]
              n372 = Build Path(base path=w336, name or relative path="config" ("名称或相对路径")) -> (appended path=w334:path)
              n373 = Build Path(base path=w334, name or relative path="bordII_config" ("名称或相对路径")) -> (appended path=w332:path)
              n374 = local write "配置文件目录"(w332) -> ()
            }
            frame #1 {
              # "遍历配置文件目录"
              n375 = local read "配置文件目录"() -> (w338:path)
              n376 = call "罗列目录配置文件.vi"("路径"=w338) -> ("数组"=w339:string[])  [unwired: 10 in]
              n377 = property on="加载配置文件列表" class="Ring (严格)"("Strings []"=w339) -> ()  [unwired: 2 in, 2 out]
            }
            frame #2 {
              n378 = property on="加载配置文件列表" class="Ring (严格)"() -> ("RingText.Text"=w340:string)  [unwired: 2 in, 2 out]
              n379 = local write "加载文件名称"(w340) -> ()
            }
            frame #3 {
              # "待读取配置文件路径"
              n380 = local read "配置文件目录"() -> (w342:path)
              n381 = property on="加载文件名称" class="Str"() -> ("Text.Text"=w341:string)  [unwired: 2 in, 2 out]
              n382 = Build Path(base path=w342, name or relative path=w341) -> (appended path=w343:path)
              n383 = local write "配置文件路径"(w343) -> ()
            }
            frame #4 {
              # "读取默认配置的配置内容"
              n384 = local read "配置文件路径"() -> (w345:path)
              n385 = call "函数测试配置文件读取.vi"("配置文件路径"=w345) -> ("D_IN_1"=w344:string[][])  [unwired: 6 in, 3 out]
              n386 = local write "D_IN_1"(w344) -> ()
            }
          }
        }
        frame #1 {
          n387 = for {
            N: 32 ("维数大小") -> [_]
            tunnel: [w386] -> w350 mode=indexing
            tunnel: [w382] -> w349 mode=indexing
            tunnel: [w380] -> w348 mode=indexing
            tunnel: [w377] -> w347 mode=indexing
            tunnel: [w374] -> w346 mode=indexing
            tunnel: [w371] -> w352 mode=indexing
            tunnel: [w368] -> w353 mode=indexing
            tunnel: [w365] -> w354 mode=indexing
            tunnel: [w362] -> w355 mode=indexing
            tunnel: [w357] -> w356 mode=indexing
            i -> [w359]
            n388 = local read "D_IN_1"() -> (w360:string[][])
            n389 = Index Array(array=w360, index (row)=w359, index (col)=0 ("禁用的索引 (列)")) -> (element=w386:string)
            n390 = Index Array(array=w360, index (row)=w359, index (col)=2 ("禁用的索引 (列)")) -> (element=w376:string)
            n391 = Index Array(array=w360, index (row)=w359, index (col)=3 ("禁用的索引 (列)")) -> (element=w372:string)
            n392 = Index Array(array=w360, index (row)=w359, index (col)=4 ("禁用的索引 (列)")) -> (element=w370:string)
            n393 = Index Array(array=w360, index (row)=w359, index (col)=5 ("禁用的索引 (列)")) -> (element=w367:string)
            n394 = Index Array(array=w360, index (row)=w359, index (col)=9 ("禁用的索引 (列)")) -> (element=w358:string)
            n395 = Index Array(array=w360, index (row)=w359, index (col)=1 ("禁用的索引 (列)")) -> (element=w379:string)
            n396 = Index Array(array=w360, index (row)=w359, index (col)=6 ("禁用的索引 (列)")) -> (element=w363:string)
            n397 = Index Array(array=w360, index (row)=w359, index (col)=7 ("禁用的索引 (列)")) -> (element=w383:string)
            n398 = Index Array(array=w360, index (row)=w359, index (col)=8 ("禁用的索引 (列)")) -> (element=w381:string)
            n399 = Decimal String To Number(string=w376) -> (number=w374:i32)  [unwired: 2 in, 1 out]
            n400 = Decimal String To Number(string=w372) -> (number=w371:i32)  [unwired: 2 in, 1 out]
            n401 = Decimal String To Number(string=w370) -> (number=w368:i32)  [unwired: 2 in, 1 out]
            n402 = Decimal String To Number(string=w379) -> (number=w377:i32)  [unwired: 2 in, 1 out]
            n403 = Fract/Exp String To Number(string=w367) -> (number=w365:dbl)  [unwired: 3 in, 1 out]
            n404 = Fract/Exp String To Number(string=w358) -> (number=w357:dbl)  [unwired: 3 in, 1 out]
            n405 = Fract/Exp String To Number(string=w363) -> (number=w362:dbl)  [unwired: 3 in, 1 out]
            n406 = Fract/Exp String To Number(string=w383) -> (number=w382:dbl)  [unwired: 3 in, 1 out]
            n407 = Fract/Exp String To Number(string=w381) -> (number=w380:dbl)  [unwired: 3 in, 1 out]
          }
          n408 = global write "试验配置信息.vi" "名称"(w350) -> ()
          n409 = global write "试验配置信息.vi" "设定输入通道"(w346) -> ()
          n410 = global write "试验配置信息.vi" "输出切换ID"(w352) -> ()
          n411 = global write "试验配置信息.vi" "输入切换ID"(w353) -> ()
          n412 = global write "试验配置信息.vi" "参数A1"(w354) -> ()
          n413 = global write "试验配置信息.vi" "允许误差"(w356) -> ()
          n414 = global write "试验配置信息.vi" "设定输出通道"(w347) -> ()
          n415 = global write "试验配置信息.vi" "参数A2"(w355) -> ()
          n416 = global write "试验配置信息.vi" "min"(w349) -> ()
          n417 = global write "试验配置信息.vi" "Max"(w348) -> ()
        }
        frame #2 {
          n418 = for {
            N: 32 -> [_]
            i -> [w391]
            w395 = 5 ("num")
            n419 = global read "试验配置信息.vi" "名称"() -> (w394:string[])
            n420 = global read "试验配置信息.vi" "Max"() -> (w398:dbl[])
            n421 = global read "试验配置信息.vi" "min"() -> (w399:dbl[])
            n422 = Index Array(array=w399, index=w391) -> (element=w397:dbl)
            n423 = Index Array(array=w398, index=w391) -> (element=w396:dbl)
            n424 = for {
              N: w395 -> [_]
              tunnel: w391 -> [w410]
              tunnel: w397 -> [w407]
              tunnel: w396 -> [w406]
              tunnel: w395 -> [w405]
              i -> [w403]
              n425 = call "等分取数据.vi"("Max"=w406, "MIN"=w407, "num"=w405) -> ("数据点"=w404:dbl[])  [unwired: 5 in]
              n426 = Add(x=2, y=w403) -> (x+y=w408:i32)
              n427 = local read "Analog_IN"() -> (w412:string[][])
              n428 = Index Array(array=w404, index=w403) -> (element=w401:dbl)
              n429 = Number To Fractional String(number=w401, precision (6)=i16 3 ("精度(6)")) -> (F-format string=w402:string)  [unwired: 2 in]
              n430 = Replace Array Subset(array=w412, new element=w402, index (row)=w410, index (col)=w408) -> (w411:string[][])
              n431 = local write "Analog_IN"(w411) -> ()
            }
            n432 = Index Array(array=w394, index=w391) -> (element=w389:string)
            n433 = local read "Analog_IN"() -> (w392:string[][])
            n434 = Replace Array Subset(array=w392, new element=w389, index (row)=w391, index (col)=1) -> (w393:string[][])
            n435 = local write "Analog_IN"(w393) -> ()
          }
        }
        frame #3 {
          n436 = for {
            N: 32 -> [_]
            i -> [w415]
            n437 = for {
              N: 6 -> [_]
              tunnel: w415 -> [w422]
              i -> [w419]
              n438 = Quotient & Remainder(x=w422, y=2) -> (x-y*floor(x/y)=w420:i32)  [unwired: 1 out]
              n439 = Equal To 0?(x=w420) -> (x = 0?=w423:bool)
              n440 = case shown="假" w423 {
                tunnel: [u32 16448250 u32 15723488] -> w416
                frame False {
                }
                frame True {
                }
              }
              n441 = Bundle(w422, w419) -> (w418:cluster{i32, i32})  [unwired: 1 in]
              n442 = property on="Analog_WC" class="Tbl (严格)"("Active Cell"=w418) -> (error out=w417:errorcluster)  [unwired: 2 in, 1 out]
              n443 = property on="Analog_WC" class="Tbl (严格)"(error in=w417, "Cell BG Color"=w416) -> ()  [unwired: 1 in, 2 out]
            }
          }
        }
      }
      n444 = local write "同步_1"(0 ("同步_2")) -> ()
      n445 = local write "退出？"(FALSE ("退出？")) -> ()
      n446 = Initialize Array(FALSE, 32 ("维数大小"), 5 ("维数大小")) -> (w328:bool[][])
      n447 = Initialize Array(FALSE, 32 ("维数大小")) -> (w316:bool[])
      n448 = property on="Analog_back" class="Tbl (严格)"("DisabledEnum"=T1."Disabled" ("禁用")) -> ()  [unwired: 2 in, 2 out]
      n449 = local write "数组_选择"(w316) -> ()
      n450 = local write "合格？"(w328) -> ()
      n451 = Initialize Array(0.0, 32 ("维数大小"), 5 ("维数大小")) -> (w319:dbl[][])
      n452 = local write "数组_设定值"(w319) -> ()
      n453 = Initialize Array("", 32 ("维数大小"), 5 ("维数大小")) -> (w323:string[][])
      n454 = local write "Analog_back"(w323) -> ()
      n455 = local write "Analog_WC"(w323) -> ()
      n456 = local write "第几组数据"(w312) -> ()
      n457 = local write "第几个数据"(w312) -> ()
    }
  }
  n458 = Obtain Notifier(name (unnamed)=w8, notification data type=w8) -> (notifier out=w10:refnum<notifier>, error out=w9:errorcluster)  [unwired: 2 in, 1 out]
  n459 = while {
    tunnel: w10 -> [w431]
    tunnel: w9 -> [w430]
    tunnel: [w429] -> w7
    tunnel: [w428] -> w6
    stop <- w433 stop-if-true
    n460 = Wait Until Next ms Multiple(millisecond multiple=u32 10 ("毫秒倍数")) -> ()  [unwired: 1 out]
    n461 = Wait on Notification(notifier=w431, timeout in ms (-1)=20 ("超时毫秒(-1)"), error in (no error)=w430) -> (notifier out=w429:refnum<notifier>, notification=w435:string, error out=w428:errorcluster)  [unwired: 1 in, 1 out]
    n462 = Equal?(x=w435, y="DSP" ("通知")) -> (x = y?=w426:bool)
    n463 = case shown="真" w426 {
      frame False {
      }
      frame True {
        n464 = stacked-sequence {
          frame #0 {
            n465 = for {
              N: 32 -> [_]
              i -> [w438]
              n466 = local read "数组_选择"() -> (w439:bool[])
              n467 = local read "数组_设定值"() -> (w440:dbl[][])
              n468 = Index Array(array=w439, index=w438) -> (element=w437:bool)
              n469 = case shown="真" w437 {
                tunnel: w438 -> [_ w441]
                tunnel: w440 -> [_ w443]
                frame False {
                }
                frame True {
                  n470 = Increment(x=w441) -> (x+1=w444:i32)
                  n471 = To Unsigned Byte Integer(number=w444) -> (unsigned 8bit integer=w445:u8)
                  n472 = call "一组模拟量CAN切换开关.vi"("第几组数据"=w445) -> ()  [unwired: 10 in, 1 out]
                  n473 = case shown="真" TRUE {
                    tunnel: w441 -> [_ w446]
                    tunnel: w443 -> [_ w447]
                    frame False {
                    }
                    frame True {
                      n474 = local write "第几组数据"(w446) -> ()
                      n475 = for {
                        N: 5 -> [_]
                        tunnel: w446 -> [w451]
                        tunnel: w447 -> [w450]
                        i -> [w449]
                        n476 = while {
                          tunnel: w451 -> [w459]
                          tunnel: w450 -> [w458]
                          tunnel: w449 -> [w457]
                          stop <- w454 stop-if-true
                          n477 = local read "同步_1"() -> (w455:i32)
                          n478 = Wait Until Next ms Multiple(millisecond multiple=u32 10 ("毫秒倍数")) -> ()  [unwired: 1 out]
                          n479 = Equal?(x=w455, y=0) -> (x = y?=w456:bool)
                          n480 = case shown="真" w456 {
                            tunnel: w459 -> [_ w464]
                            tunnel: w458 -> [_ w463]
                            tunnel: w457 -> [_ w462]
                            tunnel: [FALSE w461] -> w454
                            frame False {
                            }
                            frame True {
                              n481 = stacked-sequence {
                                tunnel: w464 -> [w472 _ _]
                                tunnel: w463 -> [w469 _ _]
                                tunnel: w462 -> [w467 _ _]
                                tunnel: [_ _ w484] -> w461
                                frame #0 {
                                # "PCI板卡下发模拟量数据"
                                n482 = global read "试验配置信息.vi" "设定输出通道"() -> (w471:i32[])
                                n483 = To Long Integer(number=w472) -> (32bit integer=w468:i32)
                                n484 = local write "第几个数据"(w467) -> ()
                                n485 = Index Array(array=w469, index (row)=w468, index (col)=w467) -> (element=w465:dbl)
                                n486 = Index Array(array=w471, index=w468) -> (element=w470:i32)
                                n487 = case shown="1" w470 {
                                tunnel: [w476 w479] -> w466
                                tunnel: w465 -> [w474 w477]
                                frame 0, Default {
                                n488 = Build Array(w474, 0.0) -> (w476:dbl[])
                                }
                                frame 1 {
                                n489 = Build Array(0.0, w477) -> (w479:dbl[])
                                }
                                }
                                n490 = call "Convert to Dynamic Data"("Array"=w466) -> ("Dynamic Data Type"=w473:dynamicdata)  [unwired: 3 out]
                                n491 = call "DAQNavi Assistant"("data in(DDT)"=w473) -> ()  [unwired: 2 in, 17 out]
                                }
                                frame #1 {
                                w483 = "ANumCheck" ("名称（未命名）")
                                n492 = Obtain Notifier(name (unnamed)=w483, notification data type=w483) -> (notifier out=w482:refnum<notifier>)  [unwired: 2 in, 2 out]
                                n493 = local write "同步_1"(1 ("y")) -> ()
                                n494 = Send Notification(notification="NumCheck" ("通知"), notifier=w482) -> ()  [unwired: 1 in, 2 out]
                                }
                                frame #2 {
                                n495 = local read "同步_1"() -> (w486:i32)
                                n496 = Equal?(x=w486, y=1) -> (x = y?=w484:bool)
                                }
                              }
                            }
                          }
                        }
                      }
                    }
                  }
                }
              }
            }
          }
          frame #1 {
            n497 = property on="btn_取消" class="Bool"("DisabledEnum"=T1."Enabled" ("禁用")) -> ()  [unwired: 2 in, 2 out]
          }
        }
      }
    }
    n498 = local read "退出？"() -> (w433:bool)
  }
  n499 = Release Notifier(notifier=w7, error in (no error)=w6) -> ()  [unwired: 1 in, 3 out]
  n500 = Obtain Notifier(name (unnamed)=w5, notification data type=w5) -> (notifier out=w4:refnum<notifier>, error out=w3:errorcluster)  [unwired: 2 in, 1 out]
  n501 = while {
    tunnel: w4 -> [w494]
    tunnel: w3 -> [w493]
    tunnel: [w492] -> w2
    tunnel: [w491] -> w1
    stop <- w490 stop-if-true
    n502 = Wait Until Next ms Multiple(millisecond multiple=u32 10 ("毫秒倍数")) -> ()  [unwired: 1 out]
    n503 = Wait on Notification(notifier=w494, timeout in ms (-1)=20 ("超时毫秒(-1)"), error in (no error)=w493) -> (notifier out=w492:refnum<notifier>, notification=w496:string, error out=w491:errorcluster)  [unwired: 1 in, 1 out]
    n504 = Equal?(x=w496, y="NumCheck" ("通知")) -> (x = y?=w488:bool)
    n505 = case shown="真" w488 {
      frame False {
      }
      frame True {
        n506 = call "DAQNavi Assistant2"() -> ("error out"=w501:errorcluster, "data out(DDT)"=w502:dynamicdata)  [unwired: 2 in, 16 out]
        n507 = Unbundle By Name(w501) -> ("status"=w499:bool)
        n508 = case shown="真" w499 {
          frame False {
          }
          frame True {
            n509 = call "超时"() -> ()  [unwired: 10 in, 2 out]
            n510 = local write "同步_1"(0 ("同步_1")) -> ()
          }
        }
        n511 = call "从动态数据转换"("Dynamic Data Type"=w502) -> ("Array"=w503:dbl[])  [unwired: 3 in]
        n512 = To Single Precision Float(number=w503) -> (single precision float=w498:sgl[])
        n513 = Not(x=w499) -> (.not. x?=w500:bool)
        n514 = case shown="真" w500 {
          tunnel: w498 -> [_ w505]
          frame False {
          }
          frame True {
            n515 = stacked-sequence {
              tunnel: w505 -> [w531 _ _ _ _]
              frame #0 {
                n516 = global read "试验配置信息.vi" "设定输入通道"() -> (w530:i32[])
                n517 = local read "第几组数据"() -> (w529:i32)
                n518 = local read "第几组数据"() -> (w516:i32)
                n519 = global read "试验配置信息.vi" "允许误差"() -> (w517:dbl[])
                n520 = global read "试验配置信息.vi" "参数A1"() -> (w525:dbl[])
                n521 = global read "试验配置信息.vi" "参数A2"() -> (w524:dbl[])
                n522 = global read "试验配置信息.vi" "Max"() -> (w518:dbl[])
                n523 = global read "试验配置信息.vi" "min"() -> (w519:dbl[])
                n524 = local read "第几个数据"() -> (w527:i32)
                n525 = local read "数组_设定值"() -> (w541:dbl[][])
                n526 = Index Array(array=w530, index=w529) -> (element=w528:i32)
                n527 = Index Array(array=w531, index=w528) -> (element=w507:sgl)
                n528 = Index Array(array=w518, index=w516) -> (element=w515:dbl)
                n529 = Index Array(array=w519, index=w516) -> (element=w514:dbl)
                n530 = Index Array(array=w525, index=w516) -> (element=w523:dbl)
                n531 = Index Array(array=w524, index=w516) -> (element=w522:dbl)
                n532 = Index Array(array=w517, index=w516) -> (element=w511:dbl)
                n533 = Subtract(x=w515, y=w514) -> (x-y=w513:dbl)
                n534 = local read "Analog_back"() -> (w535:string[][])
                n535 = local read "第几个数据"() -> (w532:i32)
                n536 = Absolute Value(x=w513) -> (abs(x)=w512:dbl)
                n537 = Index Array(array=w541, index (row)=w516, index (col)=w527) -> (element=w526:dbl)
                n538 = local read "数组_选择"() -> (w521:bool[])
                n539 = Number To Fractional String(number=w507, precision (6)=i16 3 ("精度(6)")) -> (F-format string=w506:string)  [unwired: 2 in]
                n540 = call "函数公式.vi"("参数 b"=w522, "参数 a"=w523, "设定值 1"=w526) -> ("y"=w520:dbl)  [unwired: 5 in, 1 out]
                n541 = Replace Array Subset(array=w535, new element=w506, index (row)=w529, index (col)=w532) -> (w534:string[][])
                n542 = call "误差计算.vi"("选择?"=w521, "允许误差"=w511, "模拟量量程范围"=w512, "设定值_1"=w520, "反馈值_1"=w507) -> ("字符串_误差_1"=w509:string, "合格_1?"=w510:bool)  [unwired: 4 in, 1 out]
                n543 = local write "Analog_back"(w534) -> ()
                n544 = local read "第几个数据"() -> (w533:i32)
                n545 = local read "Analog_WC"() -> (w540:string[][])
                n546 = local read "第几组数据"() -> (w538:i32)
                n547 = Replace Array Subset(array=w540, new element=w509, index (row)=w538, index (col)=w533) -> (w539:string[][])
                n548 = local read "合格？"() -> (w536:bool[][])
                n549 = local write "Analog_WC"(w539) -> ()
                n550 = Replace Array Subset(array=w536, new element=w510, index (row)=w538, index (col)=w533) -> (w537:bool[][])
                n551 = local write "合格？"(w537) -> ()
              }
              frame #1 {
                n552 = local read "合格？"() -> (w546:bool[][])
                n553 = local read "第几组数据"() -> (w543:i32)
                n554 = Index Array(array=w546, index (row)=w543) -> (element=w548:bool[])  [unwired: 1 in]
                n555 = And Array Elements(Boolean array=w548) -> (logical AND=w545:bool)
                n556 = local read "数组_选择"() -> (w544:bool[])
                n557 = Index Array(array=w544, index=w543) -> (element=w542:bool)
                n558 = case shown="真" w542 {
                  tunnel: [cluster{u32, u32}[] [{12369084, 12369084}] w551] -> w547
                  tunnel: w545 -> [_ w550]
                  frame False {
                  }
                  frame True {
                    n559 = case shown="真" w550 {
                      tunnel: [cluster{u32, u32}[] [{16730410, 16711680}] cluster{u32, u32}[] [{61205, 6618880}]] -> w551
                      frame False {
                      }
                      frame True {
                      }
                    }
                  }
                }
                n560 = case shown="31" w543 {
                  tunnel: w547 -> [w554 w555 w556 w557 w558 w559 w560 w561 w562 w563 w564 w565 w566 w567 w568 w569 w570 w571 w572 w573 w574 w575 w576 w577 w578 w579 w580 w581 w582 w583 w584 w585]
                  frame 0, Default {
                    n561 = property on="light_1" class="Bool (严格)"("Colors [4]"=w554) -> ()  [unwired: 2 in, 2 out]
                  }
                  frame 1 {
                    n562 = property on="light_2" class="Bool (严格)"("Colors [4]"=w555) -> ()  [unwired: 2 in, 2 out]
                  }
                  frame 2 {
                    n563 = property on="light_3" class="Bool (严格)"("Colors [4]"=w556) -> ()  [unwired: 2 in, 2 out]
                  }
                  frame 3 {
                    n564 = property on="light_4" class="Bool (严格)"("Colors [4]"=w557) -> ()  [unwired: 2 in, 2 out]
                  }
                  frame 4 {
                    n565 = property on="light_5" class="Bool (严格)"("Colors [4]"=w558) -> ()  [unwired: 2 in, 2 out]
                  }
                  frame 5 {
                    n566 = property on="light_6" class="Bool (严格)"("Colors [4]"=w559) -> ()  [unwired: 2 in, 2 out]
                  }
                  frame 6 {
                    n567 = property on="light_7" class="Bool (严格)"("Colors [4]"=w560) -> ()  [unwired: 2 in, 2 out]
                  }
                  frame 7 {
                    n568 = property on="light_8" class="Bool (严格)"("Colors [4]"=w561) -> ()  [unwired: 2 in, 2 out]
                  }
                  frame 8 {
                    n569 = property on="light_9" class="Bool (严格)"("Colors [4]"=w562) -> ()  [unwired: 2 in, 2 out]
                  }
                  frame 9 {
                    n570 = property on="light_10" class="Bool (严格)"("Colors [4]"=w563) -> ()  [unwired: 2 in, 2 out]
                  }
                  frame 10 {
                    n571 = property on="light_11" class="Bool (严格)"("Colors [4]"=w564) -> ()  [unwired: 2 in, 2 out]
                  }
                  frame 11 {
                    n572 = property on="light_12" class="Bool (严格)"("Colors [4]"=w565) -> ()  [unwired: 2 in, 2 out]
                  }
                  frame 12 {
                    n573 = property on="light_13" class="Bool (严格)"("Colors [4]"=w566) -> ()  [unwired: 2 in, 2 out]
                  }
                  frame 13 {
                    n574 = property on="light_14" class="Bool (严格)"("Colors [4]"=w567) -> ()  [unwired: 2 in, 2 out]
                  }
                  frame 14 {
                    n575 = property on="light_15" class="Bool (严格)"("Colors [4]"=w568) -> ()  [unwired: 2 in, 2 out]
                  }
                  frame 15 {
                    n576 = property on="light_16" class="Bool (严格)"("Colors [4]"=w569) -> ()  [unwired: 2 in, 2 out]
                  }
                  frame 16 {
                    n577 = property on="light_17" class="Bool (严格)"("Colors [4]"=w570) -> ()  [unwired: 2 in, 2 out]
                  }
                  frame 17 {
                    n578 = property on="light_18" class="Bool (严格)"("Colors [4]"=w571) -> ()  [unwired: 2 in, 2 out]
                  }
                  frame 18 {
                    n579 = property on="light_19" class="Bool (严格)"("Colors [4]"=w572) -> ()  [unwired: 2 in, 2 out]
                  }
                  frame 19 {
                    n580 = property on="light_20" class="Bool (严格)"("Colors [4]"=w573) -> ()  [unwired: 2 in, 2 out]
                  }
                  frame 20 {
                    n581 = property on="light_21" class="Bool (严格)"("Colors [4]"=w574) -> ()  [unwired: 2 in, 2 out]
                  }
                  frame 21 {
                    n582 = property on="light_22" class="Bool (严格)"("Colors [4]"=w575) -> ()  [unwired: 2 in, 2 out]
                  }
                  frame 22 {
                    n583 = property on="light_23" class="Bool (严格)"("Colors [4]"=w576) -> ()  [unwired: 2 in, 2 out]
                  }
                  frame 23 {
                    n584 = property on="light_24" class="Bool (严格)"("Colors [4]"=w577) -> ()  [unwired: 2 in, 2 out]
                  }
                  frame 24 {
                    n585 = property on="light_25" class="Bool (严格)"("Colors [4]"=w578) -> ()  [unwired: 2 in, 2 out]
                  }
                  frame 25 {
                    n586 = property on="light_26" class="Bool (严格)"("Colors [4]"=w579) -> ()  [unwired: 2 in, 2 out]
                  }
                  frame 26 {
                    n587 = property on="light_27" class="Bool (严格)"("Colors [4]"=w580) -> ()  [unwired: 2 in, 2 out]
                  }
                  frame 27 {
                    n588 = property on="light_28" class="Bool (严格)"("Colors [4]"=w581) -> ()  [unwired: 2 in, 2 out]
                  }
                  frame 28 {
                    n589 = property on="light_29" class="Bool (严格)"("Colors [4]"=w582) -> ()  [unwired: 2 in, 2 out]
                  }
                  frame 29 {
                    n590 = property on="light_30" class="Bool (严格)"("Colors [4]"=w583) -> ()  [unwired: 2 in, 2 out]
                  }
                  frame 30 {
                    n591 = property on="light_31" class="Bool (严格)"("Colors [4]"=w584) -> ()  [unwired: 2 in, 2 out]
                  }
                  frame 31 {
                    n592 = property on="light_32" class="Bool (严格)"("Colors [4]"=w585) -> ()  [unwired: 2 in, 2 out]
                  }
                }
              }
              frame #2 {
                n593 = local read "第几组数据"() -> (w587:i32)
                n594 = local read "第几个数据"() -> (w590:i32)
                n595 = local read "合格？"() -> (w591:bool[][])
                n596 = local read "数组_选择"() -> (w589:bool[])
                n597 = Index Array(array=w591, index (row) #1=w587, index (col) #1=w590, index (col) #2=w590) -> (element #1=w588:bool)  [unwired: 1 in, 1 out]
                n598 = Index Array(array=w589, index=w587) -> (element=w586:bool)
                n599 = case shown="真" w586 {
                  tunnel: w590 -> [_ w595]
                  tunnel: w588 -> [_ w594]
                  tunnel: w587 -> [_ w593]
                  frame False {
                  }
                  frame True {
                    n600 = call "误差表格颜色.vi"("合格？"=w594, "第几组"=w593) -> ("颜色"=w592:u32)  [unwired: 9 in]
                    n601 = Bundle("第几组数据"=w593, "第几个数据"=w595) -> (w597:cluster{"第几组数据":i32, "第几个数据":i32})  [unwired: 1 in]
                    n602 = property on="Analog_WC" class="Tbl (严格)"("Active Cell"=w597) -> (error out=w596:errorcluster)  [unwired: 2 in, 1 out]
                    n603 = property on="Analog_WC" class="Tbl (严格)"(error in=w596, "Cell BG Color"=w592) -> ()  [unwired: 1 in, 2 out]
                  }
                }
              }
              frame #3 {
                n604 = Wait Until Next ms Multiple(millisecond multiple=u32 100 ("毫秒倍数")) -> ()  [unwired: 1 out]
              }
              frame #4 {
                n605 = local write "同步_1"(0 ("同步_1")) -> ()
              }
            }
          }
        }
      }
    }
    n606 = local read "退出？"() -> (w490:bool)
  }
  n607 = Release Notifier(notifier=w2, error in (no error)=w1) -> ()  [unwired: 1 in, 3 out]
